vi "Configure Spurious Emission (Segment Frequency Setup).vi"(0 "VISA resource name":refnum<visa-resource-name>, 5 "Spurious Start Frequency":dbl[](array[numeric]) min=-100000000.0 max=43099999700.0, 7 "Spurious Stop Frequency":dbl[](array[numeric]) min=-100000000.0 max=43100000000.0, 11 "error in (no error)":errorcluster) -> (4 "VISA resource name out":refnum<visa-resource-name>, 15 "error out":errorcluster)   [LabVIEW 2020, in "Anritsu Signal Analyzer Series.lvlib"]
doc: "Configures the frequency for segment parameter of Spurious Emission measurement."
uses:
  Anritsu Signal Analyzer Series.lvlib
panel:
  # "Hz"
  # "Hz"
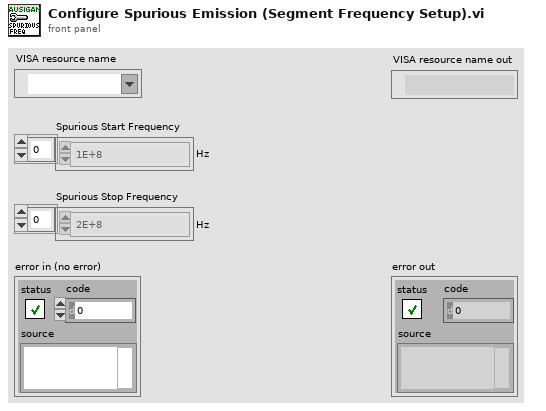
[diagram p1: front panel]
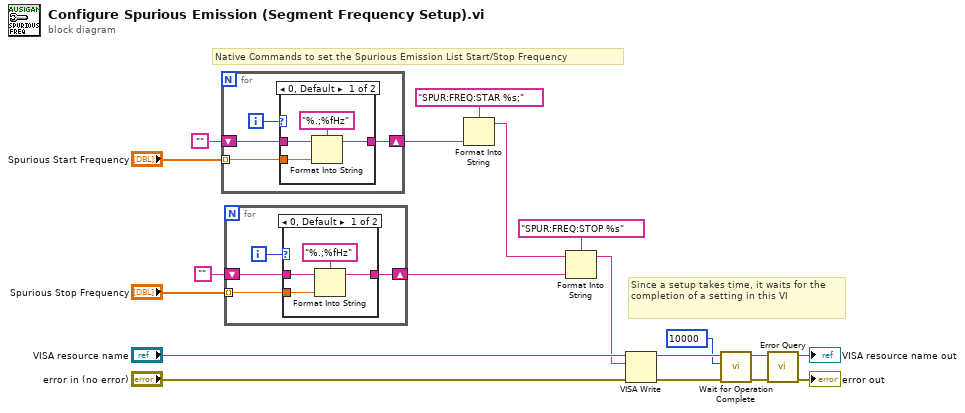
[diagram p0: block diagram]
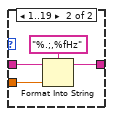
[diagram p2: hidden frame]
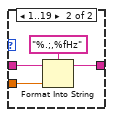
[diagram p3: hidden frame]
diagram:
  # "Since a setup takes time, it waits for the completion of a setting in this VI"
  # "Native Commands to set the Spurious Emission List Start/Stop Frequency"
  n1 = for {
    shift-right: [w20] -> w8
    shift-left: "" -> [w22]
    tunnel: "Spurious Start Frequency" -> [w21] mode=indexing
    i -> [w23]
    n2 = case shown="0, Default" w23 {
      tunnel: w22 -> [w26 w29]
      tunnel: [w24 w28] -> w20
      tunnel: w21 -> [w25 w30]
      frame 0, Default {
        n3 = Format Into String(format string="%.;%fHz" ("string"), initial string=w26, w25) -> (resulting string=w24:string)  [unwired: 1 in, 1 out]
      }
      frame 1..19 {
        n4 = Format Into String(format string="%.;,%fHz" ("string"), initial string=w29, w30) -> (resulting string=w28:string)  [unwired: 1 in, 1 out]
      }
    }
  }
  n5 = for {
    shift-right: [w32] -> w6
    shift-left: "" -> [w34]
    tunnel: "Spurious Stop Frequency" -> [w33] mode=indexing
    i -> [w35]
    n6 = case shown="0, Default" w35 {
      tunnel: w34 -> [w38 w41]
      tunnel: [w36 w40] -> w32
      tunnel: w33 -> [w37 w42]
      frame 0, Default {
        n7 = Format Into String(format string="%.;%fHz" ("string"), initial string=w38, w37) -> (resulting string=w36:string)  [unwired: 1 in, 1 out]
      }
      frame 1..19 {
        n8 = Format Into String(format string="%.;,%fHz" ("string"), initial string=w41, w42) -> (resulting string=w40:string)  [unwired: 1 in, 1 out]
      }
    }
  }
  n9 = Format Into String(format string="SPUR:FREQ:STAR %s;" ("_CommandSet"), w8) -> (resulting string=w11:string)  [unwired: 2 in, 1 out]
  n10 = Format Into String(format string="SPUR:FREQ:STOP %s" ("_CommandSet"), initial string=w11, w6) -> (resulting string=w10:string)  [unwired: 1 in, 1 out]
  n11 = VISA Write(VISA resource name="VISA resource name", write buffer=w10, error in (no error)="error in (no error)") -> (VISA resource name out=w3:refnum<visa-resource-name>, error out=w2:errorcluster)  [unwired: 1 out]
  n12 = call "Wait for Operation Complete.vi"("error in (no error)"=w2, "Maximum Time (10000mSec)"=10000, "VISA resource name"=w3) -> ("error out"=w4:errorcluster, "VISA resource name out"=w5:refnum<visa-resource-name>)  [unwired: 7 in]
  n13 = call "Error Query.vi"("error in (no error)"=w4, "VISA resource name"=w5) -> ("error out"=→"error out":errorcluster, "VISA resource name out"=→"VISA resource name out":refnum<visa-resource-name>)  [unwired: 6 in, 2 out]
